vi "SetCurrent.vi"(3 "Current":u16 step=1, 4 "error in":errorcluster, 5 "connection ID in":refnum<k5>) -> (0 "False":bool, 1 "error out":errorcluster, 2 "connection ID out":refnum<k5>)   [LabVIEW 2013]
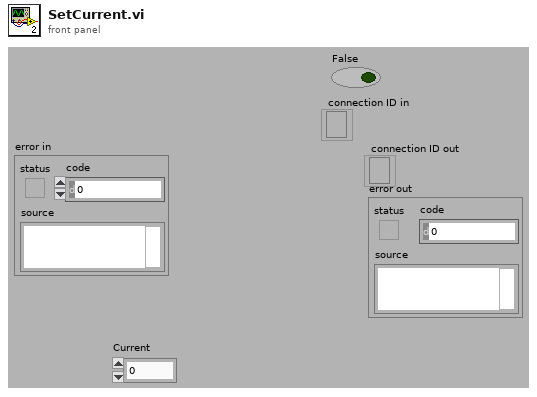
[diagram p1: front panel]
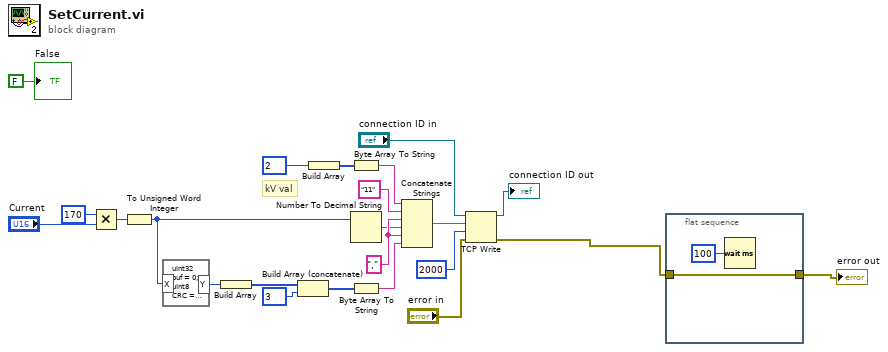
[diagram p0: block diagram]
diagram:
  w13 = "," ("string")
  # "kV val"
  n1 = Multiply(x=u16 170, y="Current") -> (x*y=w9:u16)
  n2 = To Unsigned Word Integer(number=w9) -> (unsigned 16bit integer=w8:u16)
  n3 = formula code="uInt32 buf = 0;\nuInt8 CRC = 0;\nuInt8 Y = 0;\n\nbuf = 0x31 + 0x31  + X + 0x2C;\nbuf = ~ buf;\nbuf = buf & 0x000000FF;\nCRC = buf;\nCRC &= 0x7F;\nCRC |= 0x40;\nCRC++;\nY = CRC;"("X"=w8) -> ("Y"=w12:u8)
  n4 = Build Array(w12) -> (w11:u8[])
  n5 = Build Array (concatenate)(w11, u8 3 ("y")) -> (w18:u8[])
  n6 = Build Array(u8 2 ("y")) -> (w16:u8[])
  n7 = Byte Array To String(unsigned byte array=w16) -> (string=w15:string)
  n8 = Number To Decimal String(number=w8) -> (decimal integer string=w7:string)  [unwired: 1 in]
  n9 = Byte Array To String(unsigned byte array=w18) -> (string=w10:string)
  n10 = Concatenate Strings(w15, "11" ("string"), w13, w7, w13, w10) -> (w4:string)
  n11 = TCP Write(connection ID="connection ID in", data in=w4, error in (no error)="error in", 9:2000 ("timeout ms (25000)")) -> (connection ID out=→"connection ID out":refnum<k5>, error out=w2:errorcluster)  [unwired: 1 out]
  n12 = flat-sequence {
    tunnel: [w25] -> w1
    tunnel: w2 -> [w25]
    frame #0 {
      n13 = Wait (ms)(milliseconds to wait=u32 100) -> ()  [unwired: 1 out]
    }
  }
  "error out" <- w1
  "False" <- FALSE
